vi "Handle Error.vi"(8 "error in (no error)":errorcluster, 11 "Simulated Sensor Interface Actor in":refnum<class "Simulated Sensor Interface Actor.lvclass">) -> (0 "error out":errorcluster, 2 "stop actor?":bool=TRUE, 3 "Simulated Sensor Interface Actor out":refnum<class "Simulated Sensor Interface Actor.lvclass">)   [LabVIEW 2019, in "Simulated Sensor Interface Actor.lvlib" / "Simulated Sensor Interface Actor.lvclass"]
doc: "(<B>Filename</B>: Actor Framework.lvlib:Actor.lvclass:Handle Error.vi)\n\nDefines how the actor handles an error that occurred while processing a message. By default, this method does nothing except stop the actor."
uses:
  Simulated Sensor Interface Actor.lvclass
  C:/Program Files (x86)/National Instruments/LabVIEW 2019/vi.lib/ActorFramework/Actor/Actor.lvclass
  ATM Controller/ATM Controller/Error Level.ctl
  <vilib>/ActorFramework/Actor/Actor.lvclass/Actor.ctl
  ATM Controller/ATM Controller Messages/Centrialize Error Handler Msg/Centrialize Error Handler Msg.lvclass/Centrialize Error Handler Msg.ctl
  <vilib>/ActorFramework/Message Enqueuer/Message Enqueuer.lvclass/Message Enqueuer.ctl
  <vilib>/ActorFramework/Message Enqueuer/Enqueue.vi
  ATM Controller/ATM Controller Messages/Centrialize Error Handler Msg/Centrialize Error Handler Msg.lvclass
  C:/Program Files (x86)/National Instruments/LabVIEW 2019/vi.lib/ActorFramework/Message/Message.lvclass
  <vilib>/ActorFramework/Message Priority Queue/Priority Enqueue.vi
  Sensor Interface Actor/Sensor Interface Actor/Sensor Interface Actor.lvclass
  <vilib>/ActorFramework/Actor/Actor.lvclass
  ATM Controller/ATM Controller/ATM Controller.lvclass
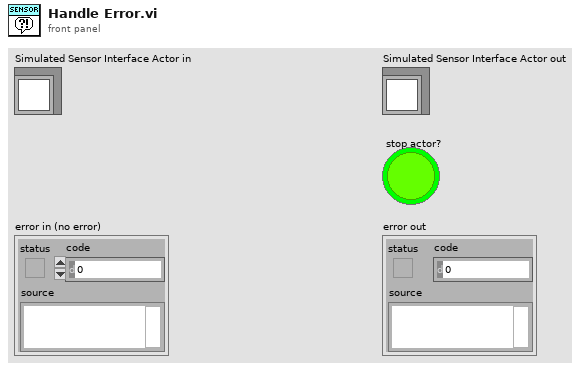
[diagram p1: front panel]
types:
  T1 = typedef "ATM Controller.lvlib/ATM Controller.lvclass/Error Level.ctl" = enum16{"Console Error", "Sensor Interface Error", "Process Step Error"}
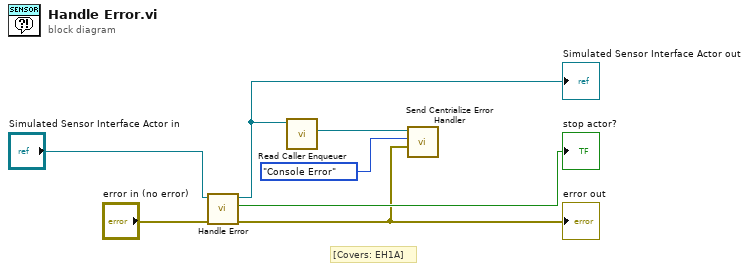
[diagram p0: block diagram]
diagram:
  # "[Covers: EH1A]"
  n1 = call-parent "Handle Error.vi"("error in (no error)"="error in (no error)", "Actor in"="Simulated Sensor Interface Actor in") -> ("error out"=w1:errorcluster, "stop actor?"=→"stop actor?":bool, "Actor out"=w4:refnum<class "Simulated Sensor Interface Actor.lvclass">)  [unwired: 7 in]
  "Simulated Sensor Interface Actor out" <- w4
  "error out" <- w1
  n2 = call <vilib>:"Read Caller Enqueuer.vi"("Actor"=w4) -> ("Caller Enqueuer"=w3:refnum<class "Message Enqueuer.lvclass">)  [unwired: 10 in]
  n3 = call "Send Centrialize Error Handler.vi"("Error"=w1, "Error Level"=Error_Level."Console Error", "Message Enqueuer"=w3) -> ()  [unwired: 7 in, 2 out]
